vi "Init_Main.vi"(8 "Error In":errorcluster) -> (0 "Error Out":errorcluster, 3 "Queue Cluster":T1)   [LabVIEW 2021, in "Queues.lvlib"]
doc: "This VI is used to create user event, create and and init the quees of the main VI and the QMH, and to create the notifier."
uses:
  Queues.lvlib
  Tipski Definicii/Main_program_queues.ctl
  Tipski Definicii/Kalibrator_Sostojbi.ctl
  Tipski Definicii/QMH_Daq_States.ctl
panel:
  # "Input"
  # "Output"
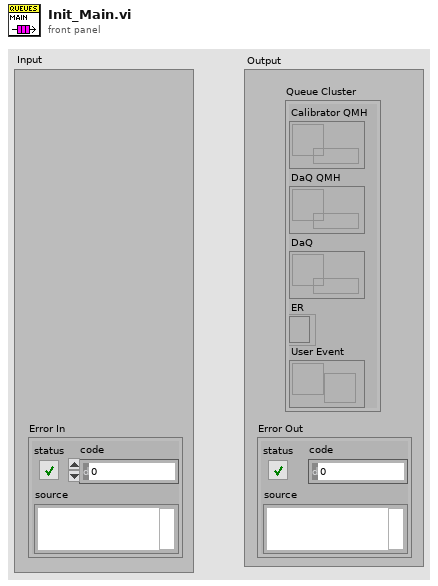
[diagram p1: front panel]
types:
  T1 = typedef "Main_program_queues.ctl" = cluster{"Calibrator QMH":refnum<queue>, "DaQ QMH":refnum<queue>, "DaQ":refnum<queue>, "ER":refnum<event-registration>, "User Event":refnum<user-event>}
  T2 = typedef "Kalibrator_Sostojbi.ctl" = enum16{"Init", "Idle", "Standby", "Operate ", "End"}
  T3 = typedef "QMH_Daq_States.ctl" = enum16{"Idle", "Start DaQ", "DaQ", "Generate Message", "Stop DaQ", "End"}
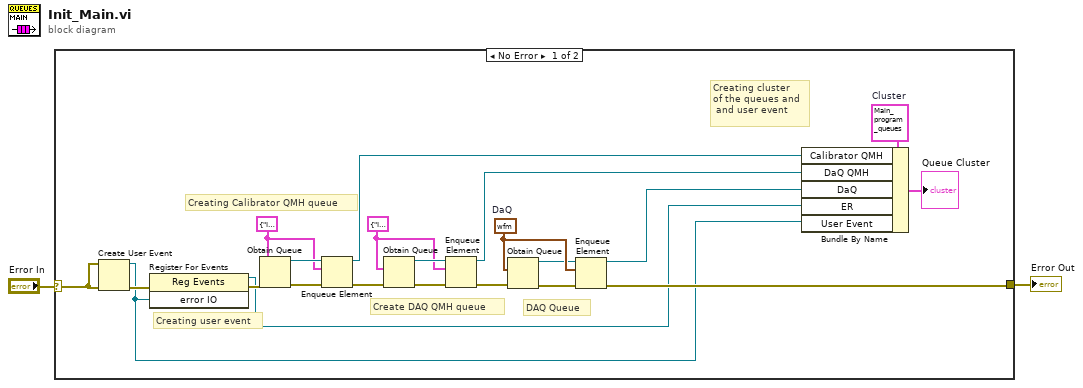
[diagram p0: block diagram]
diagram:
  n1 = case shown="No Error" "Error In" {
    selector: "Error In" -> [w20 w25]
    tunnel: [w10 w25] -> w1
    frame No Error {
      w12 = waveform(dbl) {"t0"=timestamp(0 s since 1904-01-01), "dt"=1.0, "Y"=[]}  # DaQ
      w9 = T1 {"Calibrator QMH"=refnum, "DaQ QMH"=refnum, "DaQ"=refnum, "ER"=refnum, "User Event"=refnum}  # Cluster
      w15 = cluster{"Instruction":T2, "Message":variant} {"Instruction"=enum."Init", "Message"=variant}
      w16 = cluster{"Instruction":T3, "Message":variant} {"Instruction"=enum."Idle", "Message"=variant}
      # "Creating cluster\nof the queues and\n and user event"
      # "DAQ Queue"
      # "Create DAQ QMH queue"
      # "Creating Calibrator QMH queue"
      # "Creating user event"
      n2 = Create User Event(user event datatype=w20, error in=w20) -> (user event=w3:refnum<user-event>, error out=w21:errorcluster)
      n3 = register-events(error in=w21, w3) -> (reference out=w4:refnum<event-registration>, error out=w22:errorcluster)  [unwired: 1 in]
      n4 = Obtain Queue(element data type=w15, error in (no error)=w22) -> (queue out=w24:refnum<queue>, error out=w23:errorcluster)  [unwired: 3 in, 1 out]
      n5 = Enqueue Element(queue=w24, element=w15, error in (no error)=w23) -> (queue out=w7:refnum<queue>, error out=w19:errorcluster)  [unwired: 1 in, 1 out]
      n6 = Obtain Queue(element data type=w16, error in (no error)=w19) -> (queue out=w17:refnum<queue>, error out=w18:errorcluster)  [unwired: 3 in, 1 out]
      n7 = Enqueue Element(queue=w17, element=w16, error in (no error)=w18) -> (queue out=w6:refnum<queue>, error out=w14:errorcluster)  [unwired: 1 in, 1 out]
      n8 = Obtain Queue(element data type=w12, error in (no error)=w14) -> (queue out=w11:refnum<queue>, error out=w13:errorcluster)  [unwired: 3 in, 1 out]
      n9 = Enqueue Element(queue=w11, element=w12, error in (no error)=w13) -> (queue out=w5:refnum<queue>, error out=w10:errorcluster)  [unwired: 1 in, 1 out]
      n10 = Bundle By Name(cluster=w9, "Calibrator QMH"=w7, "DaQ QMH"=w6, "DaQ"=w5, "ER"=w4, "User Event"=w3) -> (→"Queue Cluster":T1)
    }
    frame Error {
    }
  }
  "Error Out" <- w1
